vi "custom_counter_control.vi"(0 "Signal-high duration":u32=20, 1 "Signal-high lead-up":u32=10) -> ()   [LabVIEW 2015]
panel:
  out "Configuration Error messages":T1
  # "Output"
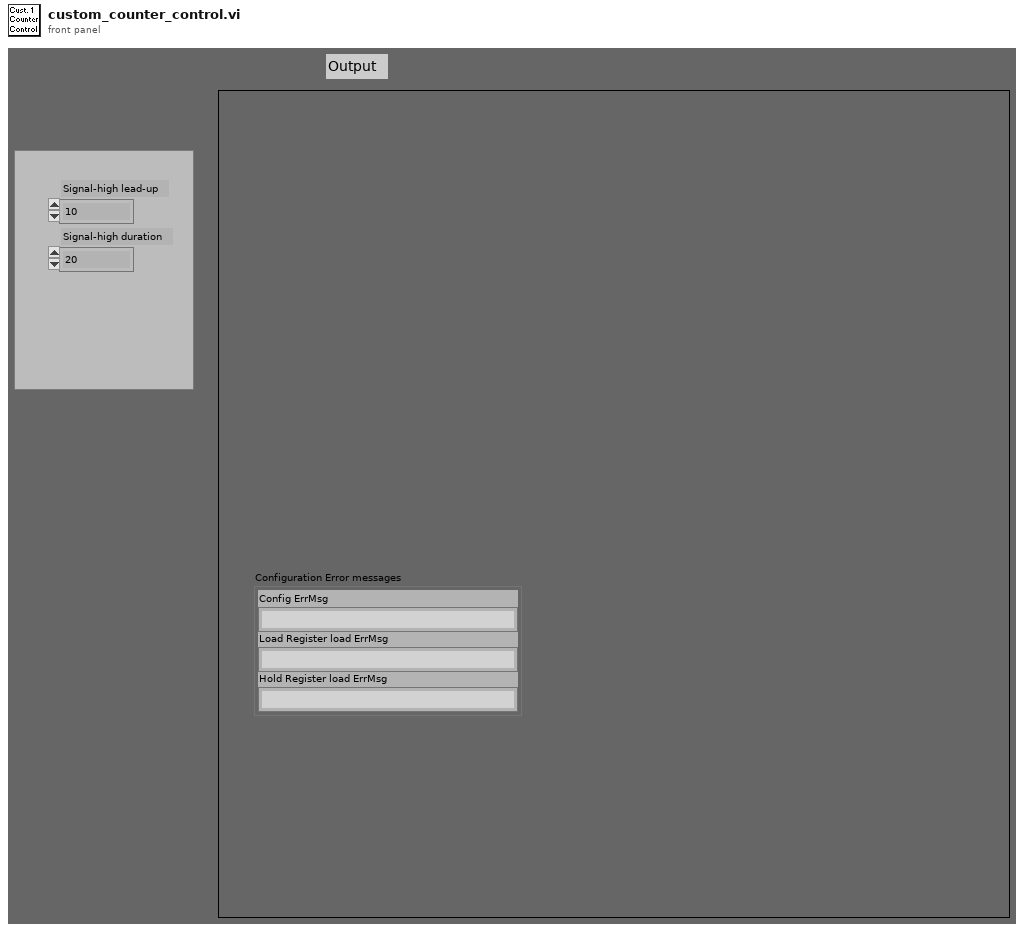
[diagram p1: front panel]
types:
  T1 = cluster{"Config ErrMsg":string, "Load Register load ErrMsg":string, "Hold Register load ErrMsg":string}
  T2 = cluster{"CounterNum":u32, "GateControl":u32, "CountSource Freq":u32, "OutputControl (LOW)":u32, "Signal-high lead-up":u32, "Signal-high duration":u32}
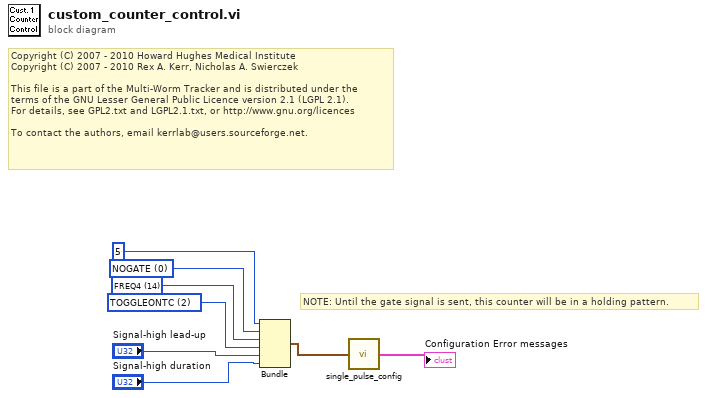
[diagram p0: block diagram]
diagram:
  w5 = u32 2 items=["ALWAYSLOW", "HIGHPULSEONTC", "TOGGLEONTC", "DISCONNECTED", "LOWPULSEONTC"] ("OutputControl (LOW)")
  w6 = u32 14 items=["TCPREVCTR", "CTRINPUT1", "CTRINPUT2", "CTRINPUT3", "CTRINPUT4", "CTRINPUT5", "GATE1", "GATE2", "GATE3", "GATE4", "GATE5", "FREQ1", "FREQ2", "FREQ3", "FREQ4", "FREQ5", "CTRINPUT6", "CTRINPUT7", "CTRINPUT8", "CTRINPUT9", "CTRINPUT10", "GATE6", "GATE7", "GATE8", "GATE9", "GATE10", "FREQ6", "FREQ7", "FREQ8", "FREQ9", "FREQ10", "CTRINPUT11", "CTRINPUT12", "CTRINPUT13", "CTRINPUT14", "CTRINPUT15", "GATE11", "GATE12", "GATE13", "GATE14", "GATE15", "FREQ11", "FREQ12", "FREQ13", "FREQ14", "FREQ15", "CTRINPUT16", "CTRINPUT17", "CTRINPUT18", "CTRINPUT19", "CTRINPUT20", "GATE16", "GATE17", "GATE18", "GATE19", "GATE20", "FREQ16", "FREQ17", "FREQ18", "FREQ19", "FREQ20"] ("CountSource Freq")
  w7 = u32 0 items=["NOGATE", "AHLTCPREVCTR", "AHLNEXTGATE", "AHLPREVGATE", "AHLGATE", "ALLGATE", "AHEGATE", "ALEGATE"] ("GateControl")
  # "Copyright (C) 2007 - 2010 Howard Hughes Medical Institute\nCopyright (C) 2007 - 2010 Rex A. Kerr, Nicholas A. Swierczek\n \nThis file is a part of the Multi-Worm Tracker and is distributed under the\nterms of the GNU Lesser General Public Licence version 2.1 (LGPL 2.1).\nFor details, see GPL2.txt and LGPL2.1.txt, or http://www.gnu.org/licences\n \nTo contact the authors, email kerrlab@users.sourceforge.net."
  # "NOTE: Until the gate signal is sent, this counter will be in a holding pattern."
  n1 = Bundle("CounterNum"=u32 5, "GateControl"=w7, "CountSource Freq"=w6, "OutputControl (LOW)"=w5, "Signal-high lead-up"="Signal-high lead-up", "Signal-high duration"="Signal-high duration") -> (w2:T2)  [unwired: 1 in]
  n2 = call "single_pulse_config.vi"("output cluster"=w2) -> ("Error output"=→"Configuration Error messages":T1)
